vi "RT_RW_2ADC_W_DACs_flatseq.vi"() -> ()   [LabVIEW 2018]
uses:
  <vilib>/FPGAPlugInAG/myRIO-1900/niLvFpga_Open_myRIO-1900.vi
  <vilib>/rvi/interface/common/dynamic/niFpgaDynamicAddResources.vi
  <vilib>/Utility/error.llb/Error Cluster From Error Code.vi
  <vilib>/rvi/errors/niLvFpgaAdjustHostInterfaceError.vi
  <vilib>/FPGAPlugInAG/Dynamic/niLvFpga_Close_Dynamic.vi
  <vilib>/rvi/interface/nirviOpenFPGA/nirviOpenFPGA.xnode
  FPGA Bitfiles/ASPE2019amplifie_FPGATarget_fpgaW&RADCsW3DAC_wVmMEUup6F8.lvbitx
  FPGA files/fpga_W&R_ADCs_W_3DAC.vi
  <vilib>/rvi/interface/nirviReadWriteControl/nirviReadWriteControl.xnode
  <vilib>/rvi/interface/nirviCloseFPGA/nirviCloseFPGA.xnode
  NiFpgaLv.dll
  <vilib>/rvi/interface/Simulation/niFpgaSimulationCallBeginRW.vi
panel:
  out "CH1 (V) 2":dbl(graph)=-0.3778018523887268
  in  "ADC 1 write":bool[](array[boolean])=[FALSE, FALSE, FALSE, FALSE, FALSE, TRUE, FALSE, FALSE, FALSE, FALSE, FALSE, FALSE, FALSE, FALSE, FALSE, FALSE]
  in  "Stop Button":bool
  in  "DAC (V)":dbl
  out "loop rate (kHz)":dbl
  in  "ADC 2 write":bool[](array[boolean])=[FALSE, FALSE, FALSE, FALSE, FALSE, TRUE, FALSE, FALSE, FALSE, FALSE, FALSE, FALSE, FALSE, FALSE, FALSE, FALSE]
  out "CH1 (V)":dbl(graph)
  # "If I change the bits on the left to CH2, signal looks noisy"
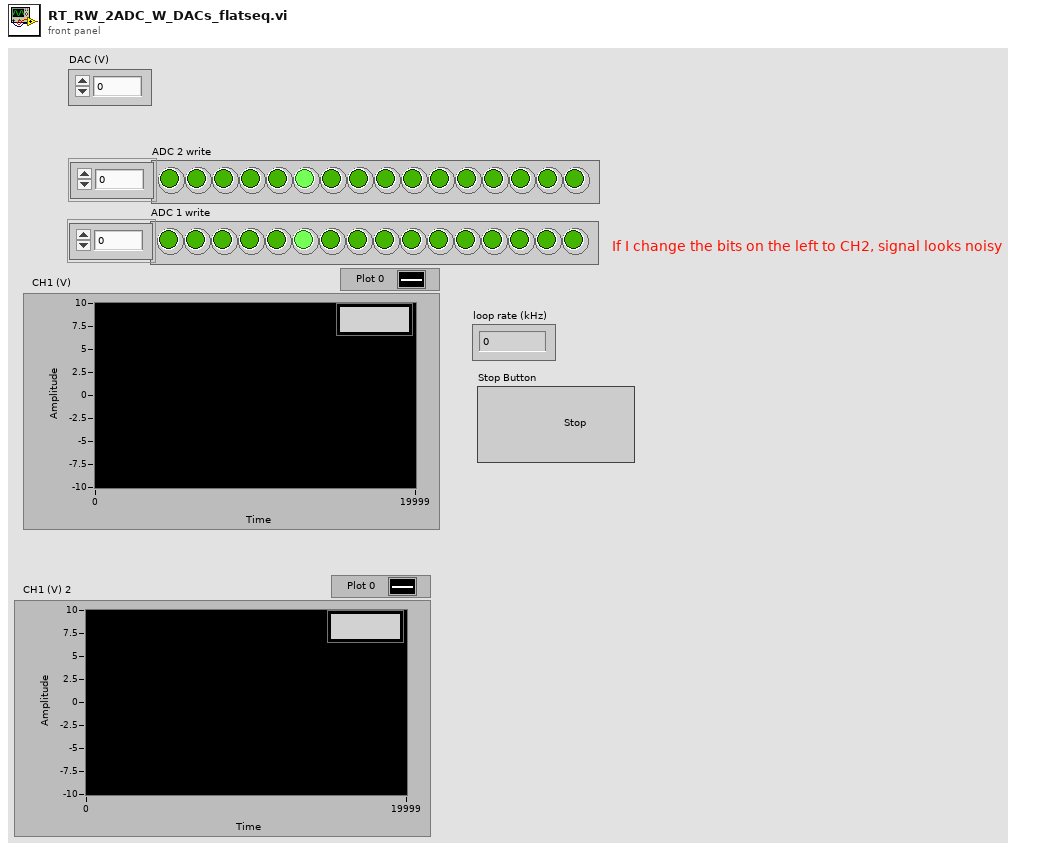
[diagram p1: front panel]
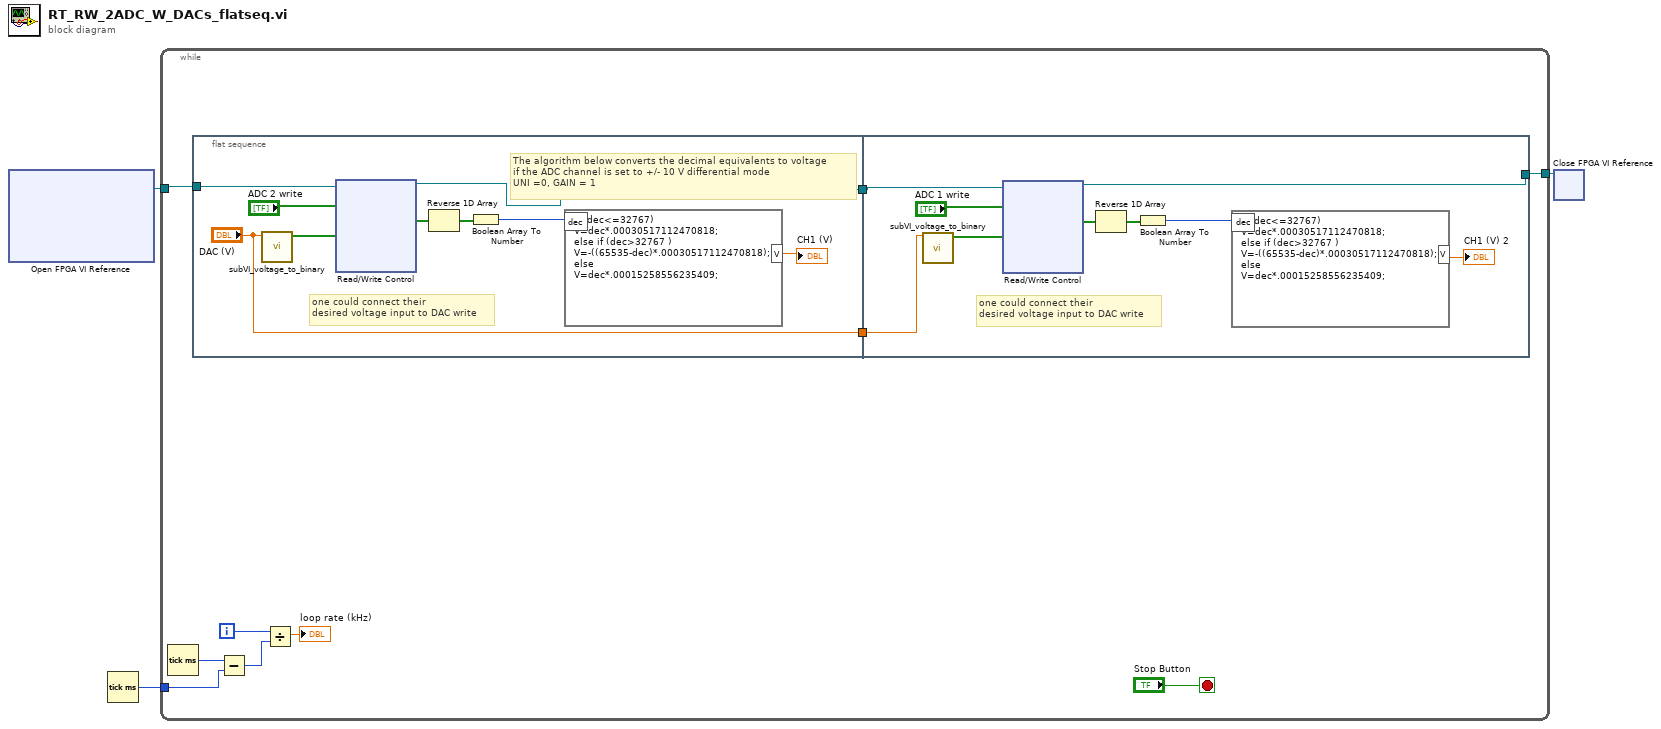
[diagram p0: block diagram]
diagram:
  n1 = xnode "Open FPGA VI Reference"() -> ("FPGA VI Reference Out"=w3:refnum<k20>)  [unwired: 2 in, 1 out]
  n2 = Tick Count (ms)() -> (millisecond timer value=w2:u32)
  n3 = while {
    tunnel: w3 -> [w13]
    tunnel: w2 -> [w10]
    tunnel: [w4] -> w1
    i -> [w9]
    stop <- "Stop Button" stop-if-true
    n4 = Tick Count (ms)() -> (millisecond timer value=w11:u32)
    n5 = flat-sequence {
      tunnel: w13 -> [w22]
      tunnel: [w17] -> w6
      tunnel: ["DAC (V)"] -> w5
      tunnel: w6 -> [w30]
      tunnel: w5 -> [w31]
      tunnel: [w23] -> w4
      frame #0 {
        # "one could connect their \ndesired voltage input to DAC write"
        # "The algorithm below converts the decimal equivalents to voltage\nif the ADC channel is set to +/- 10 V differential mode\nUNI =0, GAIN = 1"
        n6 = call "subVI_voltage_to_binary.vi"("voltage"="DAC (V)") -> ("binary"=w19:bool[])  [unwired: 10 in]
        n7 = xnode "Read/Write Control"("FPGA VI Reference In"=w22, "ADC write"="ADC 2 write", "DAC 1 write"=w19) -> ("FPGA VI Reference Out"=w17:refnum<k20>, "ADC read"=w20:bool[])  [unwired: 3 in, 1 out]
        n8 = Reverse 1D Array(array=w20) -> (reversed array=w21:bool[])
        n9 = Boolean Array To Number(Boolean array=w21) -> (number=w15:u16)
        n10 = formula code="if (dec<=32767)\nV=dec*.00030517112470818;\nelse if (dec>32767 )\nV=-((65535-dec)*.00030517112470818);\nelse\nV=dec*.00015258556235409;"("dec"=w15) -> ("V"=→"CH1 (V)":dbl)
      }
      frame #1 {
        # "one could connect their \ndesired voltage input to DAC write"
        n11 = call "subVI_voltage_to_binary.vi"("voltage"=w31) -> ("binary"=w26:bool[])  [unwired: 10 in]
        n12 = xnode "Read/Write Control"("FPGA VI Reference In"=w30, "ADC write"="ADC 1 write", "DAC 1 write"=w26) -> ("FPGA VI Reference Out"=w23:refnum<k20>, "ADC read"=w28:bool[])  [unwired: 3 in, 1 out]
        n13 = Reverse 1D Array(array=w28) -> (reversed array=w29:bool[])
        n14 = Boolean Array To Number(Boolean array=w29) -> (number=w27:u16)
        n15 = formula code="if (dec<=32767)\nV=dec*.00030517112470818;\nelse if (dec>32767 )\nV=-((65535-dec)*.00030517112470818);\nelse\nV=dec*.00015258556235409;"("dec"=w27) -> ("V"=→"CH1 (V) 2":dbl)
      }
    }
    n16 = Subtract(x=w11, y=w10) -> (x-y=w8:u32)
    n17 = Divide(x=w9, y=w8) -> (x/y=→"loop rate (kHz)":dbl)
  }
  n18 = xnode "Close FPGA VI Reference"("FPGA VI Reference In"=w1) -> ()  [unwired: 1 in, 1 out]
